vi "Read.vi"(8 "error in":errorcluster, 10 "code":string, 11 "TCP in":refnum<k5>) -> (0 "error out":errorcluster, 2 "ASCII QR Code":string, 3 "TCP Network Connection out":refnum<k5>)   [LabVIEW 2023]
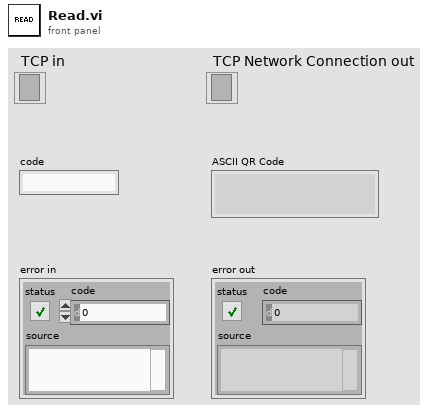
[diagram p1: front panel]
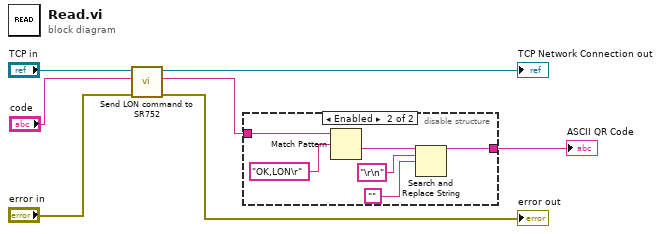
[diagram p0: block diagram]
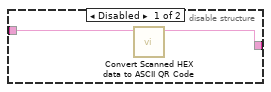
[diagram p2: hidden frame]
diagram:
  n1 = call "Send LON command to SR752.vi"("error in"="error in", "code"="code", "TCP Network Connection in"="TCP in") -> ("error out"=→"error out":errorcluster, "data out"=w2:string, "TCP Network Connection out"=→"TCP Network Connection out":refnum<k5>)  [unwired: 6 in]
  n2 = disable-structure shown="Enabled" {
    disable-tunnel: w2 -> [w9 w15]
    disable-tunnel: [w8 w12] -> w4
    frame Disabled {
      n3 = call "Convert Scanned HEX data to ASCII QR Code.vi"("Scanned HEX data"=w9) -> ("ASCII QR Code"=w8:string)  [unwired: 10 in]
    }
    frame Enabled {
      n4 = Match Pattern(string=w15, regular expression="OK,LON\r") -> (after substring=w13:string)  [unwired: 1 in, 3 out]
      n5 = Search and Replace String(input string=w13, search string="\r\n", replace string="") -> (result string=w12:string)  [unwired: 5 in, 3 out]
    }
  }
  "ASCII QR Code" <- w4
